vi "platformsupport.vi"() -> (0 "TDM Support for Platform":bool=TRUE)   [LabVIEW 2020]
panel:
  # "This is for Windows which has TDM support."
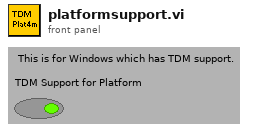
[diagram p1: front panel]
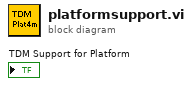
[diagram p0: block diagram]
diagram:
